vi "init connection.vi"(8 "error in (no error)":errorcluster, 9 "server port":i32, 10 "server ip":string, 11 "tcp connection in":refnum<class "tcp connection.lvclass">) -> (0 "error out":errorcluster, 3 "tcp connection out":refnum<class "tcp connection.lvclass">)   [LabVIEW 2014, in "tcp connection.lvclass"]
uses:
  tcp connection.lvclass
  typedefs/connection type.ctl
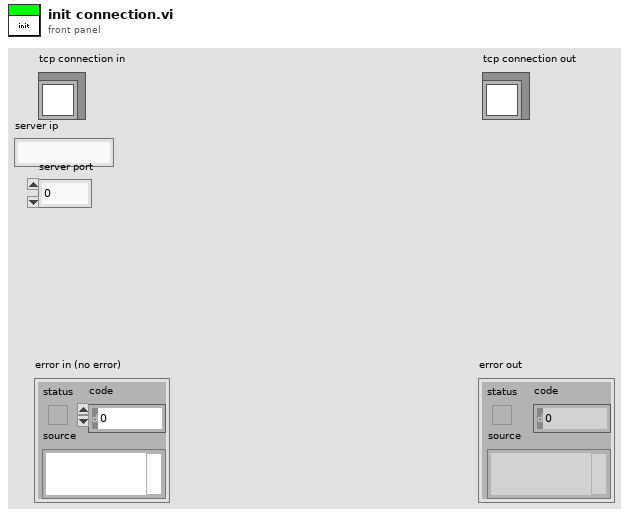
[diagram p1: front panel]
types:
  T1 = typedef "connection type.ctl" = enum16{"client", "server"}
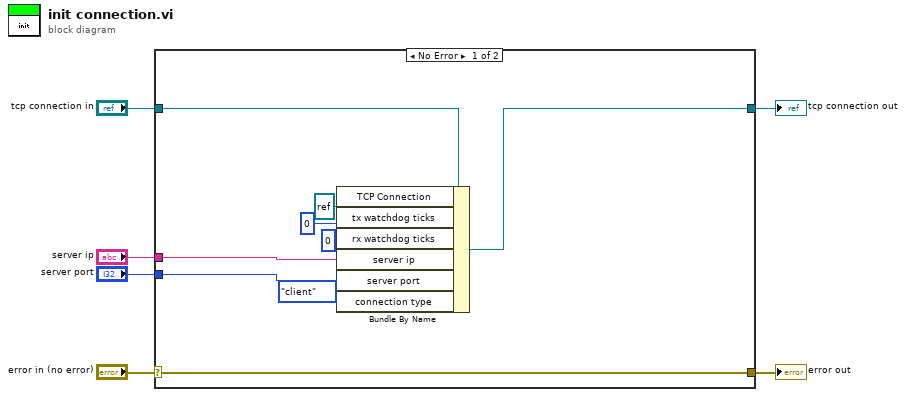
[diagram p0: block diagram]
diagram:
  n1 = case shown="No Error" "error in (no error)" {
    selector: "error in (no error)" -> [w15 w17]
    tunnel: [w15 w17] -> w5
    tunnel: [w13 w16] -> w3
    tunnel: "tcp connection in" -> [w14 w16]
    tunnel: "server ip" -> [w9 _]
    tunnel: "server port" -> [w8 _]
    frame No Error {
      n2 = Bundle By Name(cluster=w14, "TCP Connection"=refnum<k5> refnum, "tx watchdog ticks"=u32 0, "rx watchdog ticks"=u32 0, "server ip"=w9, "server port"=w8, "connection type"=connection_type."client") -> (w13:refnum<class "tcp connection.lvclass">)
    }
    frame Error {
    }
  }
  "error out" <- w5
  "tcp connection out" <- w3
